vi "Bezier length.vi"(1 "Parameters":cluster{"X":dbl, "Y":dbl}[](array[cluster])) -> (0 "Length":dbl)   [LabVIEW 2011]
doc: "This VI estimates the length of a Bézier."
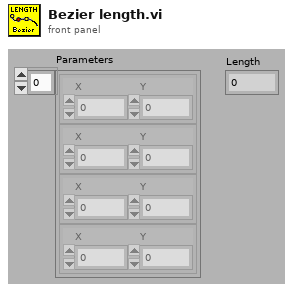
[diagram p1: front panel]
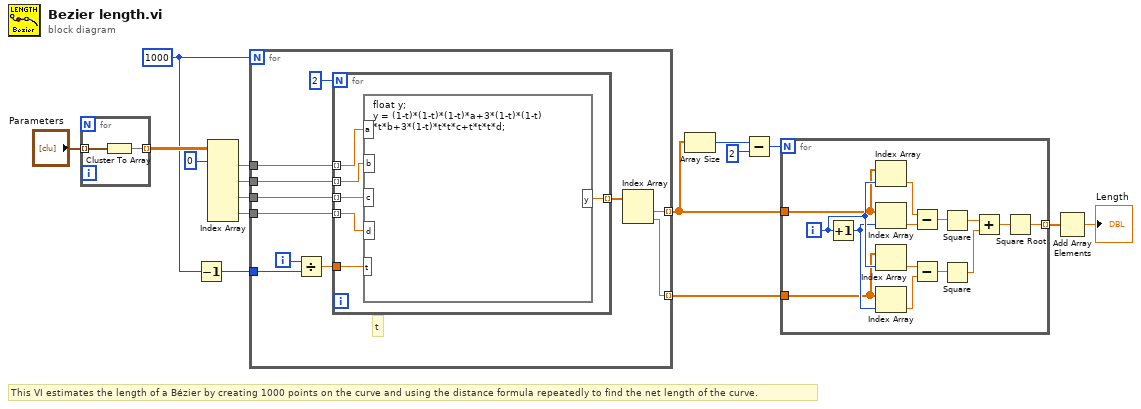
[diagram p0: block diagram]
diagram:
  w1 = 1000
  # "This VI estimates the length of a Bézier by creating 1000 points on the curve and using the distance formula repeatedly to find the net length of the curve."
  n1 = for {
    tunnel: "Parameters" -> [w18] mode=indexing
    tunnel: [w17] -> w9 mode=indexing
    n2 = Cluster To Array(cluster=w18) -> (array=w17:dbl[])
  }
  n3 = Decrement(x=w1) -> (x-1=w16:i32)
  n4 = Index Array(array=w9, index (row) #1=0 ("index (row)")) -> (element #1=w14:dbl[], element #2=w13:dbl[], element #3=w12:dbl[], element #4=w11:dbl[])  [unwired: 7 in]
  n5 = for {
    N: w1 -> [_]
    tunnel: w14 -> [w26]
    tunnel: w16 -> [w28]
    tunnel: w13 -> [w25]
    tunnel: w12 -> [w24]
    tunnel: w11 -> [w23]
    tunnel: [w21] -> w5 mode=indexing
    tunnel: [w20] -> w4 mode=indexing
    i -> [w29]
    # "t"
    n6 = Divide(x=w29, y=w28) -> (x/y=w27:dbl)
    n7 = for {
      N: 2 -> [_]
      tunnel: w27 -> [w35]
      tunnel: w26 -> [w34] mode=indexing
      tunnel: w25 -> [w33] mode=indexing
      tunnel: w24 -> [w32] mode=indexing
      tunnel: w23 -> [w31] mode=indexing
      tunnel: [w30] -> w22 mode=indexing
      n8 = formula code="float y;\ny = (1-t)*(1-t)*(1-t)*a+3*(1-t)*(1-t)\n*t*b+3*(1-t)*t*t*c+t*t*t*d;"("t"=w35, "a"=w34, "b"=w33, "c"=w32, "d"=w31) -> ("y"=w30:dbl)
    }
    n9 = Index Array(array=w22) -> (element #1=w21:dbl, element #2=w20:dbl)  [unwired: 2 in]
  }
  n10 = Array Size(array=w5) -> (size(s)=w8:i32)
  n11 = Subtract(x=w8, y=2) -> (x-y=w6:i32)
  n12 = for {
    N: w6 -> [_]
    tunnel: w5 -> [w43]
    tunnel: w4 -> [w42]
    tunnel: [w46] -> w3 mode=indexing
    i -> [w45]
    n13 = Increment(x=w45) -> (x+1=w44:i32)
    n14 = Index Array(array=w43, index=w45) -> (element=w39:dbl)
    n15 = Index Array(array=w43, index=w44) -> (element=w38:dbl)
    n16 = Index Array(array=w42, index=w45) -> (element=w41:dbl)
    n17 = Index Array(array=w42, index=w44) -> (element=w40:dbl)
    n18 = Subtract(x=w39, y=w38) -> (x-y=w37:dbl)
    n19 = Subtract(x=w41, y=w40) -> (x-y=w36:dbl)
    n20 = Square(x=w37) -> (x^2=w49:dbl)
    n21 = Square(x=w36) -> (x^2=w48:dbl)
    n22 = Add(x=w49, y=w48) -> (x+y=w47:dbl)
    n23 = Square Root(x=w47) -> (sqrt(x)=w46:dbl)
  }
  n24 = Add Array Elements(numeric array=w3) -> (sum=→"Length":dbl)
